vi "write.vi"(1 "数据输入":string, 2 "连接ID":refnum<k5>) -> (0 "连接ID输出":refnum<k5>)   [LabVIEW 2017]
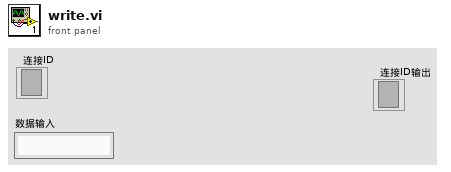
[diagram p1: front panel]
types:
  T1 = typedef "Semaphore RefNum" = refnum<k1>
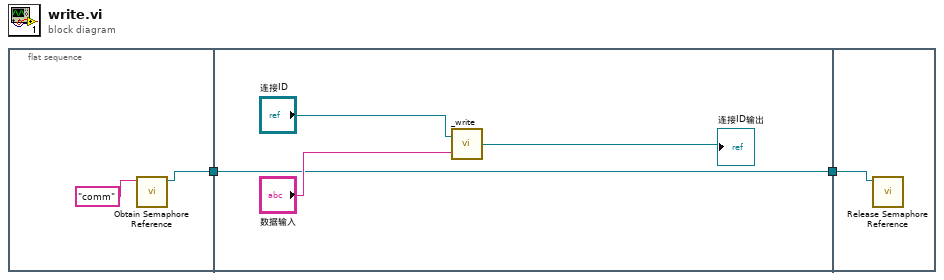
[diagram p0: block diagram]
diagram:
  n1 = flat-sequence {
    tunnel: [w3] -> w1
    tunnel: [w5] -> w2
    tunnel: w1 -> [w5]
    tunnel: w2 -> [w9]
    frame #0 {
      n2 = call <vilib>:"Obtain Semaphore Reference.vi"("name (unnamed)"="comm") -> ("semaphore"=w3:T1)  [unwired: 4 in, 2 out]
    }
    frame #1 {
      n3 = call "_write.vi"("数据输入"="数据输入", "连接ID"="连接ID") -> ("连接ID输出"=→"连接ID输出":refnum<k5>)
    }
    frame #2 {
      n4 = call <vilib>:"Release Semaphore Reference.vi"("semaphore"=w9) -> ()  [unwired: 9 in, 2 out]
    }
  }
